vi "StartMeasure.vi"(1 "error in (no error)":errorcluster) -> (0 "error IO":errorcluster caption="error out")   [LabVIEW 2018]
uses:
  InOut/Reslut.vi
panel:
  in  "任务显示":enum16{"默认", "时间波形", "光谱", "近远场"}(ring)
  out "偏振度":string
  out "偏振方向":string
  out "功率输出":string caption="功率"
  out "能量输出":string caption="能量"
  out "当前信息":string
  out "完成？":bool
  out "提示":string
  out "激光器状态":i32[](listbox)
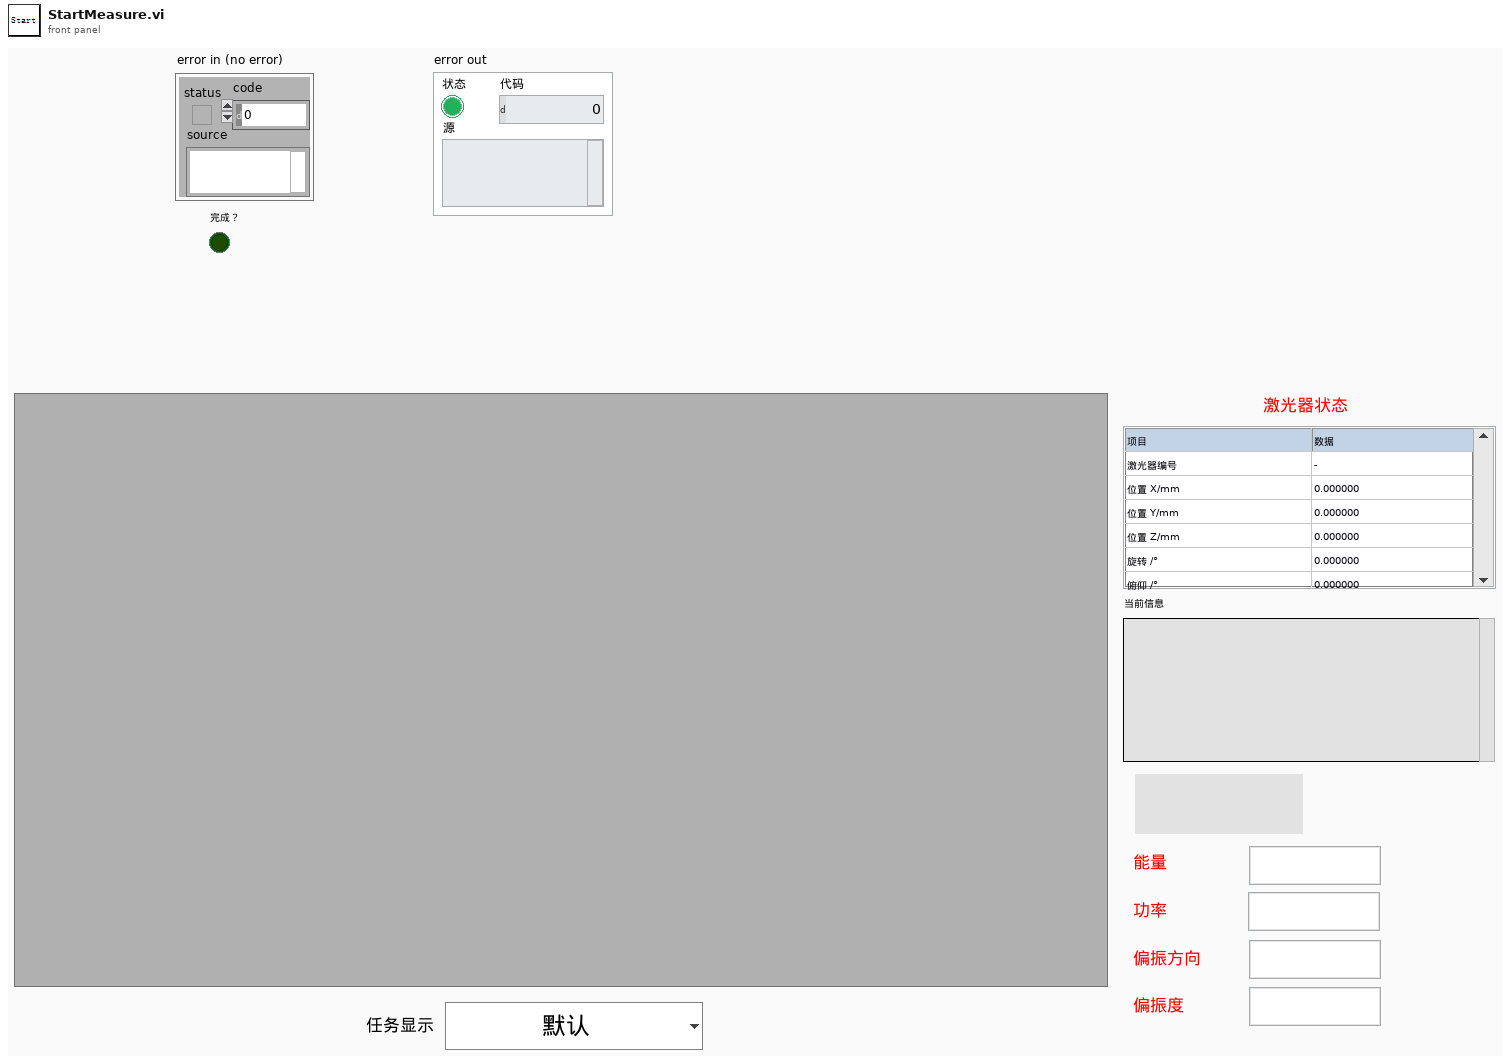
[diagram p1: front panel]
types:
  T1 = cluster{"能量计结果":string, "功率计结果":string, "能量计单位":string, " 功率计单位":string}
  T2 = cluster{"激光器型号":string, "X":dbl, "Y":dbl, "Z":dbl, "Rotate":dbl, "Pitching":dbl}
  T3 = enum8{"Enabled", "Disabled", "Disabled and Grayed Out"}
  T4 = cluster{"Selected Index []":i32[], "Selected Items":string[]}
  T5 = enum16{"功率测量", "能量测量", "光谱测量", "时间波形", "偏振测量", "近远场"}
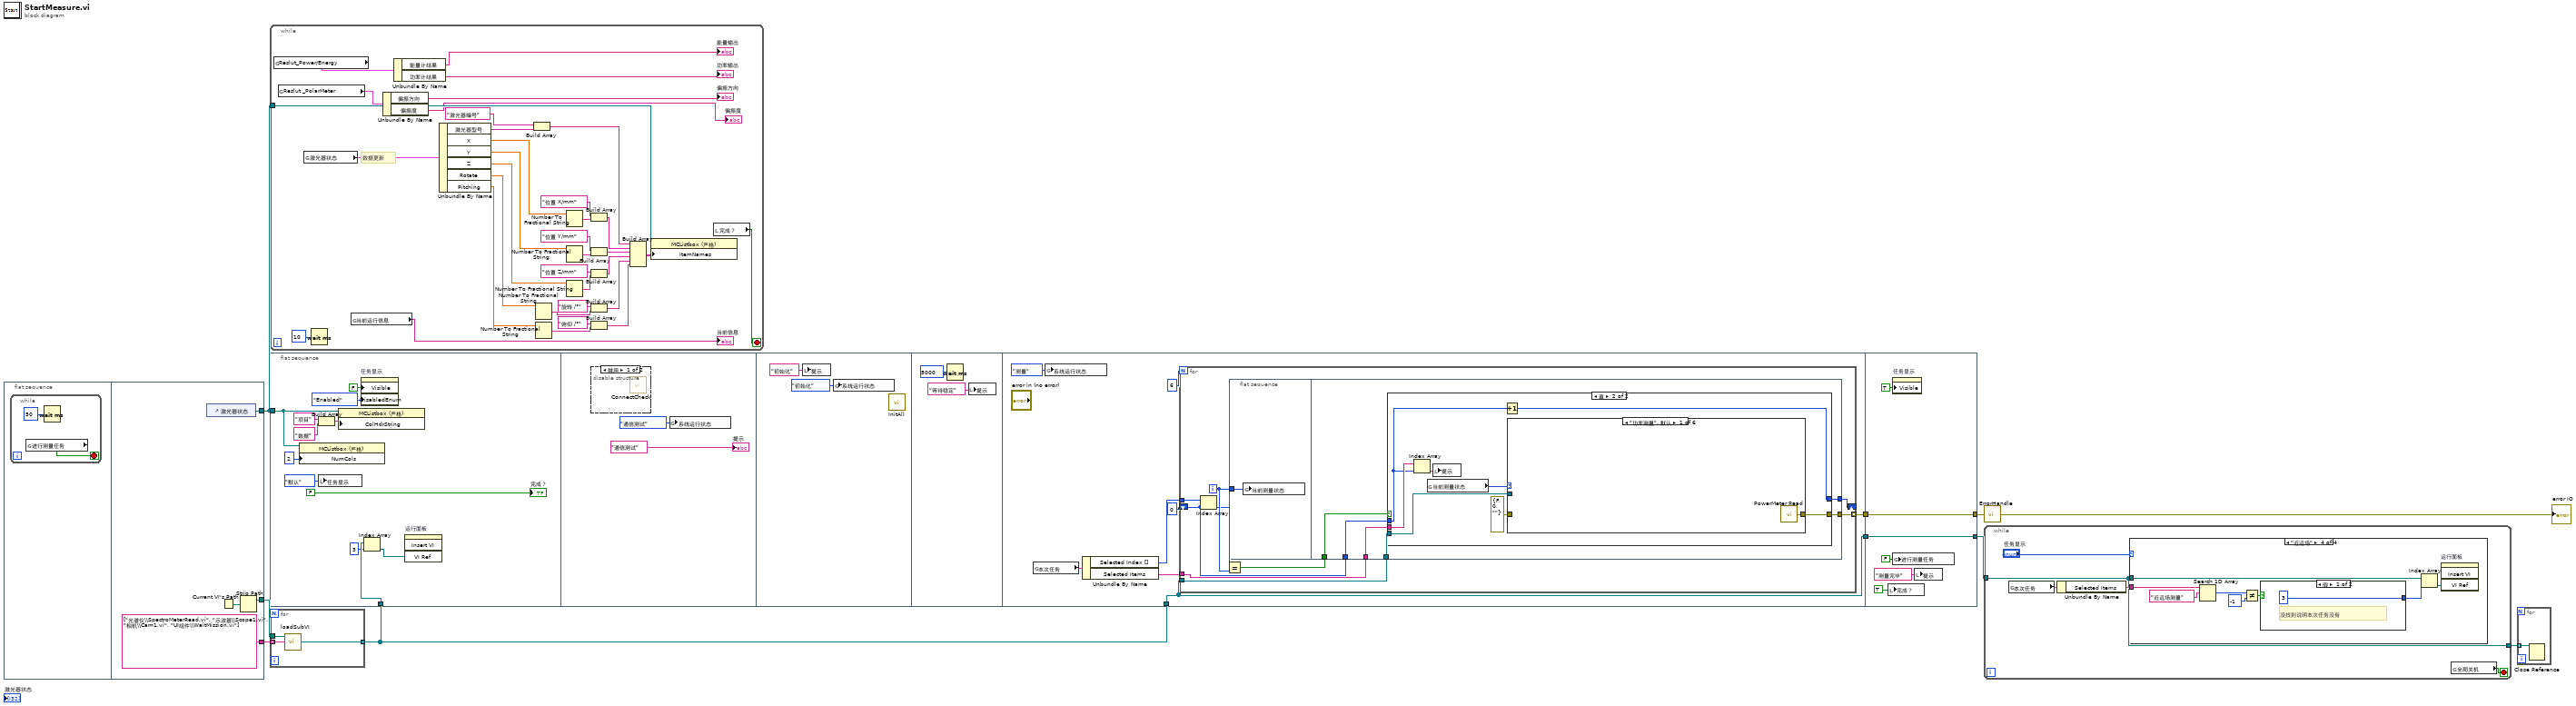
[diagram p0: block diagram]
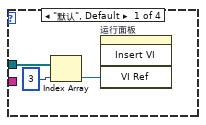
[diagram p2: hidden frame]
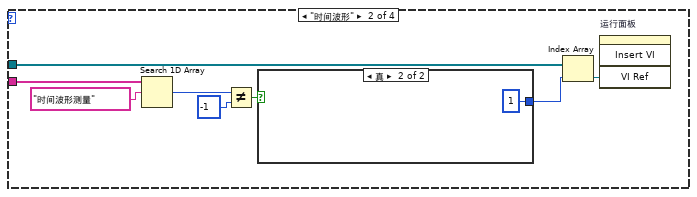
[diagram p3: hidden frame]
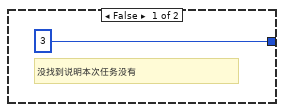
[diagram p4: hidden frame]
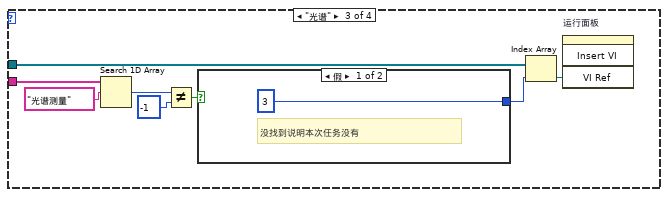
[diagram p5: hidden frame]
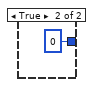
[diagram p6: hidden frame]
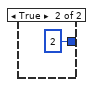
[diagram p7: hidden frame]
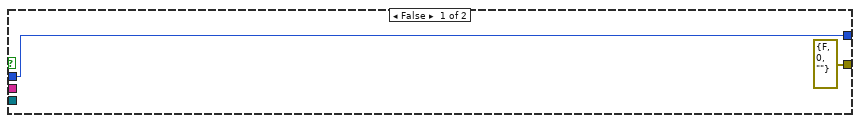
[diagram p9: hidden frame]
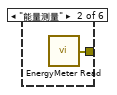
[diagram p10: hidden frame]
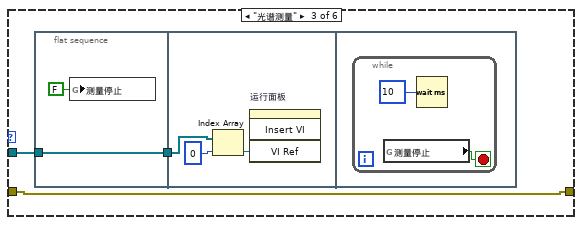
[diagram p11: hidden frame]
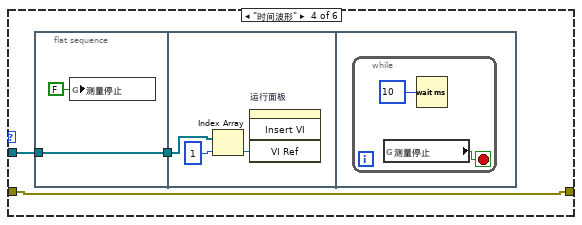
[diagram p12: hidden frame]
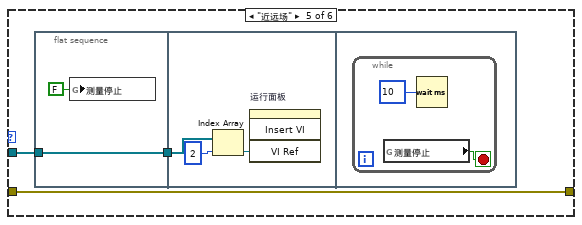
[diagram p13: hidden frame]
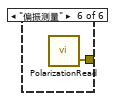
[diagram p14: hidden frame]
diagram:
  n1 = flat-sequence {
    tunnel: [w16] -> w7
    tunnel: [string[] ["光谱仪\\SpectroMeterRead.vi", "示波器\\Scope1.vi", "相机\\Cam1.vi", "UI组件\\WaitMission.vi"]] -> w6
    tunnel: [w14] -> w5
    frame #0 {
      n2 = while {
        stop <- w11 stop-if-true
        n3 = global read "参数.vi" "进行测量任务"() -> (w11:bool)
        n4 = Wait (ms)(milliseconds to wait=u32 50 ("等待时间（毫秒）")) -> ()  [unwired: 1 out]
      }
    }
    frame #1 {
      n5 = control-ref of="激光器状态"() -> (w16:refnum<vi>)
      n6 = Current VI's Path() -> (path=w13:path)
      n7 = Strip Path(path=w13) -> (stripped path=w14:path)  [unwired: 1 out]
    }
  }
  n8 = while {
    tunnel: w7 -> [w24]
    stop <- w25 stop-if-true
    # "数据更新"
    n9 = global read "Reslut.vi" "Reslut_Power/Energy"() -> (w22:T1)
    n10 = global read "Reslut.vi" "Reslut _PolarMeter"() -> (w19:cluster{" 偏振方向":string, "偏振度":string})
    n11 = global read "参数.vi" "激光器状态"() -> (w38:T2)
    n12 = Wait (ms)(milliseconds to wait=u32 10 ("等待时间（毫秒）")) -> ()  [unwired: 1 out]
    n13 = global read "globalMessage.vi" "当前运行信息"() -> (→"当前信息":string)
    n14 = Unbundle By Name(w19) -> ("偏振方向"=→"偏振方向":string, "偏振度"=→"偏振度":string)
    n15 = Unbundle By Name(w22) -> ("能量计结果"=→"能量输出":string, "功率计结果"=→"功率输出":string)
    n16 = Unbundle By Name(w38) -> ("激光器型号"=w37:string, "X"=w36:dbl, "Y"=w34:dbl, "Z"=w33:dbl, "Rotate"=w32:dbl, "Pitching"=w31:dbl)
    n17 = Build Array("激光器编号", w37) -> (w45:string[])
    n18 = Number To Fractional String(number=w32) -> (F-format string=w28:string)  [unwired: 3 in]
    n19 = Number To Fractional String(number=w31) -> (F-format string=w27:string)  [unwired: 3 in]
    n20 = Number To Fractional String(number=w36) -> (F-format string=w35:string)  [unwired: 3 in]
    n21 = Number To Fractional String(number=w34) -> (F-format string=w30:string)  [unwired: 3 in]
    n22 = Number To Fractional String(number=w33) -> (F-format string=w29:string)  [unwired: 3 in]
    n23 = Build Array("位置 X/mm", w35) -> (w44:string[])
    n24 = Build Array("位置 Y/mm", w30) -> (w43:string[])
    n25 = Build Array("位置 Z/mm", w29) -> (w42:string[])
    n26 = Build Array("旋转 /°", w28) -> (w41:string[])
    n27 = Build Array("俯仰 /°", w27) -> (w40:string[])
    n28 = Build Array(w45, w44, w43, w42, w41, w40) -> (w39:string[][])
    n29 = property on="属性节点" class="MCListbox (严格)"(reference=w24, "ItemNames"=w39) -> ()  [unwired: 1 in, 2 out]
    n30 = local read "完成？"() -> (w25:bool)
  }
  n31 = flat-sequence {
    tunnel: w7 -> [w58]
    tunnel: w1 -> [w54]
    tunnel: [w73] -> w8
    tunnel: w1 -> [w70]
    tunnel: [w70] -> w3
    tunnel: [w142] -> w10
    tunnel: w8 -> [w142]
    tunnel: w3 -> [w137]
    tunnel: [w137] -> w2
    frame #0 {
      n32 = property on="属性节点" class="MCListbox (严格)"(reference=w58, "NumCols"=u32 2 ("列数")) -> ()  [unwired: 1 in, 2 out]
      n33 = local write "任务显示"(enum16{"默认", "时间波形", "光谱", "近远场"}."默认" ("任务显示")) -> ()
      n34 = Build Array("项目", "数据") -> (w62:string[])
      n35 = property on="属性节点" class="MCListbox (严格)"(reference=w58, "ColHdrString"=w62) -> ()  [unwired: 1 in, 2 out]
      n36 = property on="任务显示" class="Enum (严格)"("Visible"=FALSE ("可见"), "DisabledEnum"=T3."Enabled" ("禁用")) -> ()  [unwired: 2 in, 2 out]
      n37 = Index Array(array=w54, index=3 ("索引")) -> (element=w52:refnum<vi>)
      n38 = invoke on="运行面板" class="SubPnl" method="Insert VI"("VI Ref"=w52) -> ()  [unwired: 3 in, 4 out]
      "完成？" <- FALSE
    }
    frame #1 {
      n39 = disable-structure shown="禁用" {
        frame Disabled {
          n40 = call "ConnectCheck.vi"() -> ()  [unwired: 12 in]
        }
        frame Enabled {
        }
      }
      n41 = global write "参数.vi" "系统运行状态"(enum16{"通信测试", "初始化", "测量", "写入"}."通信测试" ("系统运行状态")) -> ()
      "提示" <- "通信测试" ("提示")
    }
    frame #2 {
      n42 = local write "提示"("初始化" ("提示")) -> ()
      n43 = global write "参数.vi" "系统运行状态"(enum16{"通信测试", "初始化", "测量", "写入"}."初始化" ("系统运行状态")) -> ()
      n44 = call "InitAll.vi"() -> ()  [unwired: 3 in, 1 out]
    }
    frame #3 {
      n45 = Wait (ms)(milliseconds to wait=u32 5000 ("等待时间（毫秒）")) -> ()  [unwired: 1 out]
      n46 = local write "提示"("等待稳定" ("提示")) -> ()
    }
    frame #4 {
      n47 = global read "参数.vi" "本次任务"() -> (w75:T4)
      n48 = global write "参数.vi" "系统运行状态"(enum16{"通信测试", "初始化", "测量", "写入"}."测量" ("系统运行状态")) -> ()
      n49 = Unbundle By Name(w75) -> ("Selected Index []"=w74:i32[], "Selected Items"=w72:string[])
      n50 = for {
        N: 6 -> [_]
        tunnel: w74 -> [w86]
        shift-right: [w82] -> _
        shift-left: 0 -> [w80]
        tunnel: [w81] -> w73 mode=indexing
        tunnel: w72 -> [w79]
        tunnel: w70 -> [w78]
        i -> [w85]
        n51 = Index Array(array=w86, index=w80) -> (element=w83:i32)
        n52 = Equal?(x=w83, y=w85) -> (x = y?=w84:bool)
        n53 = flat-sequence {
          tunnel: w85 -> [w87]
          tunnel: w84 -> [w93]
          tunnel: w80 -> [w92]
          tunnel: [w91] -> w82
          tunnel: [w90] -> w81
          tunnel: w79 -> [w89]
          tunnel: w78 -> [w88]
          frame #0 {
            n54 = global write "参数.vi" "当前测量状态"(w87) -> ()
          }
          frame #1 {
            n55 = case shown="真" w93 {
              tunnel: w92 -> [w95 w99]
              tunnel: [w95 w103] -> w91
              tunnel: [errorcluster {"status"=FALSE, "code"=0, "source"=""} ("error out") w96] -> w90
              tunnel: w89 -> [_ w100]
              tunnel: w88 -> [_ w97]
              frame False {
              }
              frame True {
                n56 = Index Array(array=w100, index=w99) -> (element=w98:string)
                n57 = global read "参数.vi" "当前测量状态"() -> (w102:T5)
                n58 = local write "提示"(w98) -> ()
                n59 = Increment(x=w99) -> (x+1=w103:i32)
                n60 = case shown="\"功率测量\", 默认" w102 {
                  tunnel: errorcluster {"status"=FALSE, "code"=0, "source"=""} ("error out") -> [_ _ w107 w117 w127 _]
                  tunnel: w97 -> [_ _ w108 w118 w128 _]
                  tunnel: [w104 w105 w107 w117 w127 w136] -> w96
                  frame "功率测量", Default {
                    n61 = call "PowerMeter Read.vi"() -> ("错误输出"=w104:errorcluster)  [unwired: 3 in, 1 out]
                  }
                  frame "能量测量" {
                    n62 = call "EnergyMeter Read.vi"() -> ("错误输出"=w105:errorcluster)  [unwired: 3 in, 2 out]
                  }
                  frame "光谱测量" {
                    n63 = flat-sequence {
                      tunnel: w108 -> [w110]
                      tunnel: [w110] -> w106
                      tunnel: w106 -> [w113]
                      frame #0 {
                        n64 = global write "参数.vi" "测量停止"(FALSE ("测量停止")) -> ()
                      }
                      frame #1 {
                        n65 = Index Array(array=w113, index=0 ("索引")) -> (element=w111:refnum<vi>)
                        n66 = invoke on="运行面板" class="SubPnl" method="Insert VI"("VI Ref"=w111) -> ()  [unwired: 3 in, 4 out]
                      }
                      frame #2 {
                        n67 = while {
                          stop <- w115 stop-if-true
                          n68 = global read "参数.vi" "测量停止"() -> (w115:bool)
                          n69 = Wait (ms)(milliseconds to wait=u32 10 ("等待时间（毫秒）")) -> ()  [unwired: 1 out]
                        }
                      }
                    }
                  }
                  frame "时间波形" {
                    n70 = flat-sequence {
                      tunnel: w118 -> [w120]
                      tunnel: [w120] -> w116
                      tunnel: w116 -> [w123]
                      frame #0 {
                        n71 = global write "参数.vi" "测量停止"(FALSE ("测量停止")) -> ()
                      }
                      frame #1 {
                        n72 = Index Array(array=w123, index=1 ("索引")) -> (element=w121:refnum<vi>)
                        n73 = invoke on="运行面板" class="SubPnl" method="Insert VI"("VI Ref"=w121) -> ()  [unwired: 3 in, 4 out]
                      }
                      frame #2 {
                        n74 = while {
                          stop <- w125 stop-if-true
                          n75 = global read "参数.vi" "测量停止"() -> (w125:bool)
                          n76 = Wait (ms)(milliseconds to wait=u32 10 ("等待时间（毫秒）")) -> ()  [unwired: 1 out]
                        }
                      }
                    }
                  }
                  frame "近远场" {
                    n77 = flat-sequence {
                      tunnel: w128 -> [w130]
                      tunnel: [w130] -> w126
                      tunnel: w126 -> [w133]
                      frame #0 {
                        n78 = global write "参数.vi" "测量停止"(FALSE ("测量停止")) -> ()
                      }
                      frame #1 {
                        n79 = Index Array(array=w133, index=2 ("索引")) -> (element=w131:refnum<vi>)
                        n80 = invoke on="运行面板" class="SubPnl" method="Insert VI"("VI Ref"=w131) -> ()  [unwired: 3 in, 4 out]
                      }
                      frame #2 {
                        n81 = while {
                          stop <- w135 stop-if-true
                          n82 = global read "参数.vi" "测量停止"() -> (w135:bool)
                          n83 = Wait (ms)(milliseconds to wait=u32 10 ("等待时间（毫秒）")) -> ()  [unwired: 1 out]
                        }
                      }
                    }
                  }
                  frame "偏振测量" {
                    n84 = call "PolarizationRead.vi"() -> ("error IO 2"=w136:errorcluster)  [unwired: 3 in]
                  }
                }
              }
            }
          }
        }
      }
    }
    frame #5 {
      n85 = local write "完成？"(TRUE ("完成？")) -> ()
      n86 = property on="任务显示" class="Enum (严格)"("Visible"=TRUE ("可见")) -> ()  [unwired: 2 in, 2 out]
      n87 = global write "参数.vi" "进行测量任务"(FALSE ("进行测量任务")) -> ()
      n88 = local write "提示"("测量完毕" ("提示")) -> ()
    }
  }
  n89 = for {
    tunnel: w5 -> [w145]
    tunnel: w6 -> [w144] mode=indexing
    tunnel: [w143] -> w1 mode=indexing
    n90 = call "loadSubVI.vi"("VI名称"=w144, "基路径"=w145) -> ("SubVIRef"=w143:refnum<vi>)  [unwired: 2 in, 1 out]
  }
  n91 = call "ErrorHandle.vi"("Error"=w10) -> ("error IO"=→"error IO":errorcluster)
  n92 = while {
    tunnel: [w146] -> w4
    tunnel: w2 -> [w146]
    stop <- w149 stop-if-true
    n93 = global read "参数.vi" "本次任务"() -> (w148:T4)
    n94 = Unbundle By Name(w148) -> ("Selected Items"=w147:string[])
    n95 = case shown="\"近远场\"" "任务显示" {
      tunnel: w146 -> [w153 w161 w171 w180]
      tunnel: w147 -> [_ w155 w168 w175]
      frame "默认", Default {
        n96 = Index Array(array=w153, index=3 ("索引")) -> (element=w151:refnum<vi>)
        n97 = invoke on="运行面板" class="SubPnl" method="Insert VI"("VI Ref"=w151) -> ()  [unwired: 3 in, 4 out]
      }
      frame "时间波形" {
        n98 = Search 1D Array(1D array=w155, element="时间波形测量" ("元素")) -> (index of element=w158:i32)  [unwired: 1 in]
        n99 = Not Equal?(x=w158, y=-1) -> (x != y?=w156:bool)
        n100 = case shown="真" w156 {
          tunnel: [3 1 ("索引")] -> w154
          frame False {
            # "没找到说明本次任务没有"
          }
          frame True {
          }
        }
        n101 = Index Array(array=w161, index=w154) -> (element=w160:refnum<vi>)
        n102 = invoke on="运行面板" class="SubPnl" method="Insert VI"("VI Ref"=w160) -> ()  [unwired: 3 in, 4 out]
      }
      frame "光谱" {
        n103 = Search 1D Array(1D array=w168, element="光谱测量" ("元素")) -> (index of element=w166:i32)  [unwired: 1 in]
        n104 = Not Equal?(x=w166, y=-1) -> (x != y?=w164:bool)
        n105 = case shown="假" w164 {
          tunnel: [3 0 ("索引")] -> w170
          frame False {
            # "没找到说明本次任务没有"
          }
          frame True {
          }
        }
        n106 = Index Array(array=w171, index=w170) -> (element=w169:refnum<vi>)
        n107 = invoke on="运行面板" class="SubPnl" method="Insert VI"("VI Ref"=w169) -> ()  [unwired: 3 in, 4 out]
      }
      frame "近远场" {
        n108 = Search 1D Array(1D array=w175, element="近远场测量" ("元素")) -> (index of element=w178:i32)  [unwired: 1 in]
        n109 = Not Equal?(x=w178, y=-1) -> (x != y?=w176:bool)
        n110 = case shown="假" w176 {
          tunnel: [3 2 ("索引")] -> w174
          frame False {
            # "没找到说明本次任务没有"
          }
          frame True {
          }
        }
        n111 = Index Array(array=w180, index=w174) -> (element=w181:refnum<vi>)
        n112 = invoke on="运行面板" class="SubPnl" method="Insert VI"("VI Ref"=w181) -> ()  [unwired: 3 in, 4 out]
      }
    }
    n113 = global read "参数.vi" "全局关机"() -> (w149:bool)
  }
  n114 = for {
    tunnel: w4 -> [w184] mode=indexing
    n115 = Close Reference(reference=w184) -> ()  [unwired: 1 in, 1 out]
  }
